vi "RotationMatrixQuaternions.vi"(1 "Eta_q":dbl[](array[numeric])) -> (0 "R":dbl[][](array[numeric]))   [LabVIEW 2014]
uses:
  <vilib>/imath/engines/lvmath2/RunTimeEngine/IndexRead/NIMS V(S).vi
  <instcachedir>/0/NIMS V(S)_0488751826AF41519A22953C041130DC.lvgen/NIMS V(S)_0488751826AF41519A22953C041130DC_000.vi
  <vilib>/imathl/engines/lvmath/Functions/Error Handling/Create Error.vi
  <vilib>/imath/engines/lvmath2/RunTimeEngine/NodeEndStatement/NIMS_NodeEndStatement_Output.vi
  <instcachedir>/0/NIMS_NodeEndStatement_Output_53EC0D466D134D7ABD903AC30B43404B.lvgen/NIMS_NodeEndStatement_Output_53EC0D466D134D7ABD903AC30B43404B_002.vi
  <vilib>/imath/engines/lvmath2/RunTimeEngine/ErrorHandling/NIMS_Finalize Error.vi
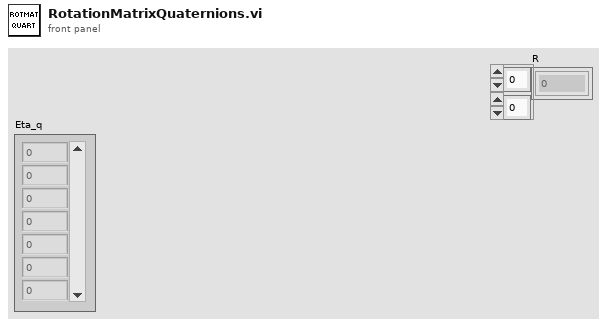
[diagram p1: front panel]
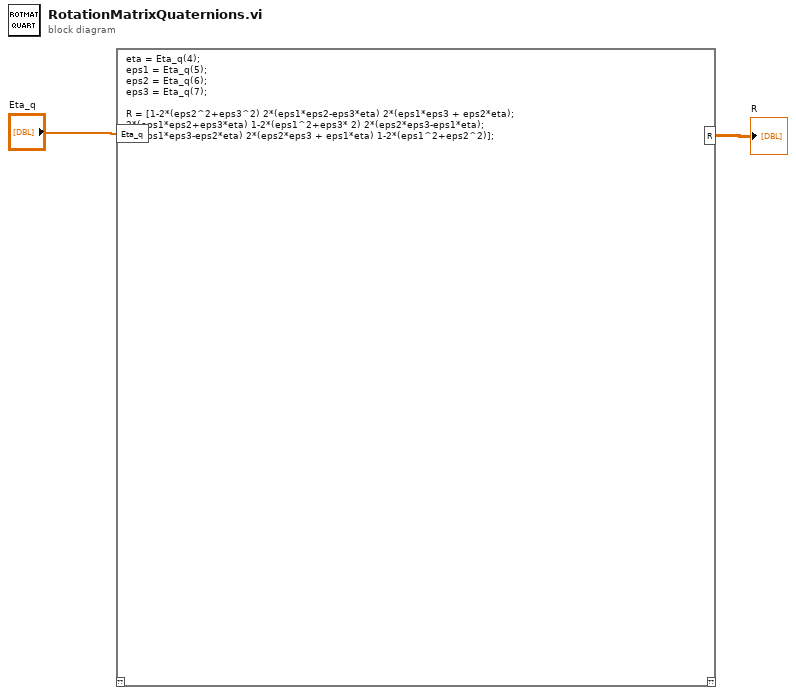
[diagram p0: block diagram]
diagram:
  n1 = mathscript code="eta = Eta_q(4);\neps1 = Eta_q(5);\neps2 = Eta_q(6);\neps3 = Eta_q(7);\n\nR = [1-2*(eps2^2+eps3^2) 2*(eps1*eps2-eps3*eta) 2*(eps1*eps3 + eps2*eta);\n2*(eps1*eps2+eps3*eta) 1-2*(eps1^2+eps3* 2) 2*(eps2*eps3-eps1*eta);\n2*(eps1*eps3-eps2*eta) 2*(eps2*eps3 + eps1*eta) 1-2*(eps1^2+eps2^2)];"("Eta_q"="Eta_q") -> ("R"=→"R":dbl[][])  [unwired: 1 in, 1 out]
